vi "Read Current Set.vi"(0 "configuration file path":path, 3 "error in (no error)":errorcluster) -> (7 "file path":path, 8 "Current Set":u8[][](array[numeric]), 10 "error out":errorcluster)   [LabVIEW 2023]
uses:
  <vilib>/Utility/config.llb/Read Key (String).vi
  <vilib>/Utility/config.llb/NI_LVConfig.lvlib
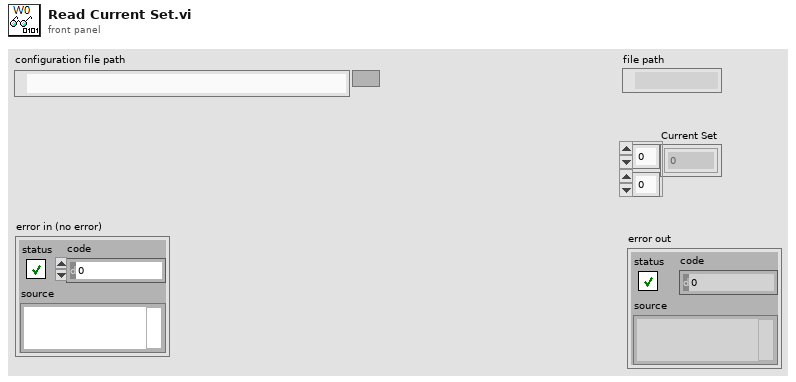
[diagram p1: front panel]
types:
  T1 = typedef "NI_LVConfig.lvlib/Config Data RefNum.ctl" = refnum<k1>
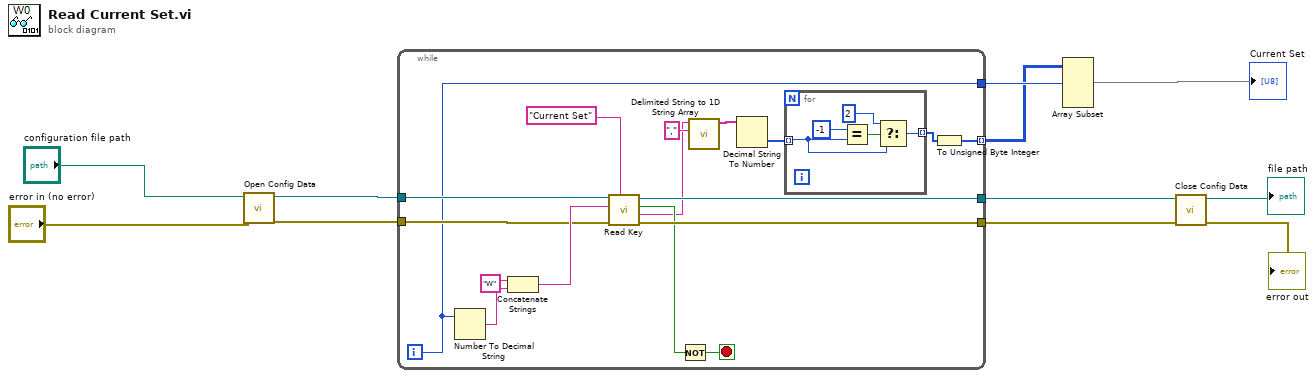
[diagram p0: block diagram]
diagram:
  n1 = call <vilib>:"Open Config Data.vi"("error in (no error)"="error in (no error)", "configuration file path"="configuration file path") -> ("error out"=w6:errorcluster, "refnum"=w7:T1)  [unwired: 7 in, 1 out]
  n2 = while {
    tunnel: [w28] -> w5
    tunnel: [w27] -> w4
    tunnel: w6 -> [w21]
    tunnel: w7 -> [w20]
    tunnel: [w19] -> w3
    tunnel: [w14] -> w2 mode=indexing
    i -> [w19]
    stop <- w22 stop-if-true
    n3 = Number To Decimal String(number=w19) -> (decimal integer string=w26:string)  [unwired: 1 in]
    n4 = Concatenate Strings("W" ("string"), w26) -> (w24:string)
    n5 = call-poly <vilib>:"Read Key.vi"("section"="Current Set", "error in (no error)"=w21, "key"=w24, "refnum"=w20) -> ("error out"=w27:errorcluster, "value"=w15:string, "found?"=w23:bool, "refnum out"=w28:T1)  [unwired: 4 in]
    n6 = Not(x=w23) -> (.not. x?=w22:bool)
    n7 = call <vilib>:"Delimited String to 1D String Array.vi"("delimiter"=",", "delimited string"=w15) -> ("string array"=w17:string[])  [unwired: 9 in]
    n8 = Decimal String To Number(string=w17) -> (number=w13:i32[])  [unwired: 2 in, 1 out]
    n9 = for {
      tunnel: w13 -> [w30] mode=indexing
      tunnel: [w29] -> w12 mode=indexing
      n10 = Equal?(x=-1, y=w30) -> (x = y?=w33:bool)
      n11 = Select(t=2 ("x"), s=w33, f=w30) -> (s? t:f=w29:i32)
    }
    n12 = To Unsigned Byte Integer(number=w12) -> (unsigned 8bit integer=w14:u8[])
  }
  n13 = Array Subset(array=w2, length (row)=w3) -> (→"Current Set":u8[][])  [unwired: 3 in]
  n14 = call <vilib>:"Close Config Data.vi"("error in (no error)"=w4, "refnum"=w5) -> ("error out"=→"error out":errorcluster, "file path"=→"file path":path)  [unwired: 8 in]
